vi "Encode.vi"(7 "Variant (Base64)":T1, 8 "error in (no error)":errorcluster, 10 "string in (not encoded)":string) -> (0 "error out":errorcluster, 2 "string out (base64-encoded)":string)   [LabVIEW 2017, in "Base64.lvlib"]
uses:
  Base64.lvlib
  Variant.ctl
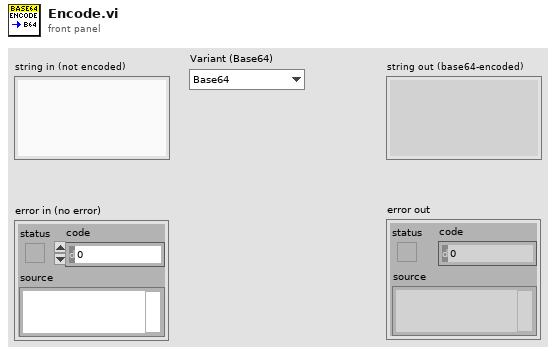
[diagram p1: front panel]
types:
  T1 = typedef "Base64.lvlib/Variant.ctl" = enum16{"Base64", "Base64-URL"}
  T2 = cluster{"unsigned byte array[0]":u8, "unsigned byte array[1]":u8, "unsigned byte array[2]":u8}
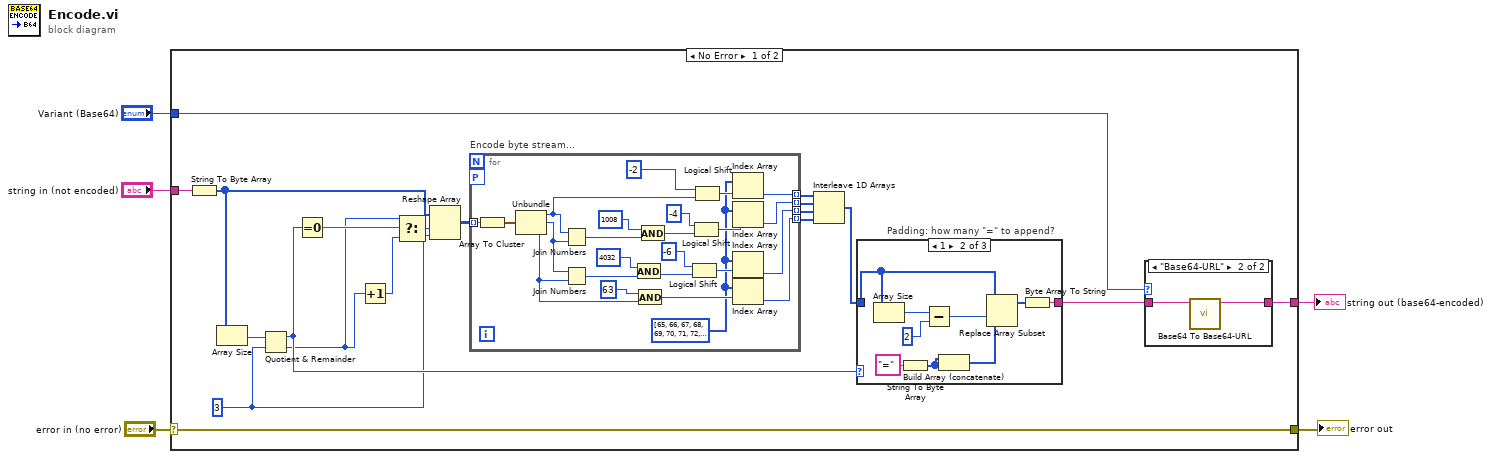
[diagram p0: block diagram]
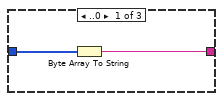
[diagram p3: hidden frame]
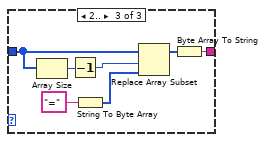
[diagram p4: hidden frame]
diagram:
  n1 = case shown="No Error" "error in (no error)" {
    selector: "error in (no error)" -> [w24 w71]
    tunnel: "string in (not encoded)" -> [w9 w70]
    tunnel: [w24 w71] -> w3
    tunnel: [w6 w70] -> w2
    tunnel: "Variant (Base64)" -> [w8 _]
    frame No Error {
      w12 = 3 ("y")
      n2 = String To Byte Array(string=w9) -> (unsigned byte array=w13:u8[])
      n3 = Array Size(array=w13) -> (size(s)=w21:i32)
      n4 = Quotient & Remainder(x=w21, y=w12) -> (x-y*floor(x/y)=w22:i32, floor(x/y)=w15:i32)
      n5 = Equal To 0?(x=w22) -> (x = 0?=w23:bool)
      n6 = Increment(x=w15) -> (x+1=w16:i32)
      n7 = Select(t=w15, s=w23, f=w16) -> (s? t:f=w11:i32)
      n8 = Reshape Array(w13, w11, w12) -> (w10:u8[][])
      n9 = for "Encode byte stream..." {
        tunnel: [w30] -> w17 mode=indexing
        tunnel: [w31] -> w18 mode=indexing
        tunnel: [w32] -> w19 mode=indexing
        tunnel: [w33] -> w20 mode=indexing
        workers-P: _ -> [_]
        tunnel: w10 -> [w28] mode=indexing
        w29 = u8[] [65, 66, 67, 68, 69, 70, 71, 72, 73, 74, 75, 76, 77, 78, 79, 80, 81, 82, 83, 84, 85, 86, 87, 88, 89, 90, 97, 98, 99, 100, 101, 102, 103, 104, 105, 106, 107, 108, 109, 110, 111, 112, 113, 114, 115, 116, 117, 118, 119, 120, 121, 122, 48, 49, 50, 51, 52, 53, 54, 55, 56, 57, 43, 47] ("unsigned byte array")
        n10 = Array To Cluster(array=w28) -> (cluster=w51:T2)
        n11 = Unbundle(w51) -> ("unsigned byte array[0]"=w40:u8, "unsigned byte array[1]"=w45:u8, "unsigned byte array[2]"=w39:u8)
        n12 = Join Numbers(hi=w40, lo=w45) -> ((hi.lo)=w49:u16)
        n13 = Join Numbers(hi=w45, lo=w39) -> ((hi.lo)=w44:u16)
        n14 = And(x=u16 4032, y=w44) -> (x .and. y?=w42:u16)
        n15 = And(x=u8 63, y=w39) -> (x .and. y?=w34:u8)
        n16 = And(x=u16 1008, y=w49) -> (x .and. y?=w47:u16)
        n17 = Logical Shift(y=i8 -6, x=w42) -> (x << y=w35:u16)
        n18 = Logical Shift(y=i8 -4, x=w47) -> (x << y=w36:u16)
        n19 = Logical Shift(y=i8 -2, x=w40) -> (x << y=w37:u8)
        n20 = Index Array(array=w29, index=w37) -> (element=w33:u8)
        n21 = Index Array(array=w29, index=w36) -> (element=w32:u8)
        n22 = Index Array(array=w29, index=w35) -> (element=w31:u8)
        n23 = Index Array(array=w29, index=w34) -> (element=w30:u8)
      }
      n24 = Interleave 1D Arrays(w20, w19, w18, w17) -> (w14:u8[])
      n25 = case "Padding: how many \"=\" to append?" shown="1" w22 {
        tunnel: [w52 w59 w68] -> w7
        tunnel: w14 -> [w53 w57 w67]
        frame ..0 {
          n26 = Byte Array To String(unsigned byte array=w53) -> (string=w52:string)
        }
        frame 1 {
          n27 = Array Size(array=w57) -> (size(s)=w58:i32)
          n28 = String To Byte Array(string="=") -> (unsigned byte array=w55:u8[])
          n29 = Subtract(x=w58, y=2) -> (x-y=w61:i32)
          n30 = Build Array (concatenate)(w55, w55) -> (w54:u8[])
          n31 = Replace Array Subset(array=w57, new element=w54, index=w61) -> (w60:u8[])
          n32 = Byte Array To String(unsigned byte array=w60) -> (string=w59:string)
        }
        frame 2.. {
          n33 = Array Size(array=w67) -> (size(s)=w63:i32)
          n34 = Decrement(x=w63) -> (x-1=w64:i32)
          n35 = String To Byte Array(string="=") -> (unsigned byte array=w65:u8[])
          n36 = Replace Array Subset(array=w67, new element=w65, index=w64) -> (w69:u8[])
          n37 = Byte Array To String(unsigned byte array=w69) -> (string=w68:string)
        }
      }
      n38 = case shown="\"Base64-URL\"" w8 {
        tunnel: w7 -> [w25 w27]
        tunnel: [w25 w26] -> w6
        frame "Base64" {
        }
        frame "Base64-URL" {
          n39 = call "Base64 To Base64-URL.vi"("Base64 String"=w27) -> ("Base64-URL String"=w26:string)  [unwired: 10 in]
        }
      }
    }
    frame Error {
    }
  }
  "string out (base64-encoded)" <- w2
  "error out" <- w3
